vi "dfd_LatticeMA_Min_FIR_C.vi"() -> ()   [LabVIEW 2017, in "NI_DigFilterTemp.lvlib"]
uses:
  <vilib>/addons/Digital Filter Design/NI_DigFilterTemp.lvlib
panel:
  in  "String":string="\n\n/* ---- Constants ----*/\n#define %CapName%_N_COEFK %kCoefKAmt%\n#define %CapName%_N_STATES %CapName%_N_COEFK\n\n/* ---- Global Variables Declaration ----*/\nstatic %CoefAType% %FilterBlkName%_CoefK[%CapName%_N_COEFK];\n%InternalFunctionsDeclaration%\n\n%ShiftDefine%\n\n%AssistantFunctions%\n\n/* ---- Implement the Fixed-Point Filter ---- */ \n%OutType% %FilterBlkName%_Filtering (%InType% sampleIn, %FilterBlkName%_State state)\n{\n\tI32 accA, accB, accTmp;\n\t%MultType% mult;\n\tint i;\n\n\taccTmp = (%I32TypeCast%sampleIn << IN2DELAY);\n\taccA = (%I32TypeCast%sampleIn << IN2SUM);\n\t\n\tfor (i = 0; i < %CapName%_N_COEFK; i++)\n\t{\n\t\t/* Filtering */\n\t\tmult = %PreMultCast%(accA << SUM2MULT);\n\t\taccB = (%FilterBlkName%_%MultA%(mult, %FilterBlkName%_CoefK[i]) << PROD2SUM);\n\t\taccB += (state[i] << DELAY2SUM);\n\t\tmult = %PreMultCast%(state[i] << DELAY2MULT);\n\t\taccA += (%FilterBlkName%_%MultA%(mult, %FilterBlkName%_CoefK[i]) << PROD2SUM);\n\n\t\t/* Update the internal states */\n\t\tstate[i] = accTmp;\n\t\taccTmp = (accB << SUM2DELAY);\n\t}\n\n\t%ApplyGainAccA%\n\n\treturn (%OutType%)accA;\n}\n\n/* ---- Internal Functions ---- */\n%InternalFunctions%\n\n/* ---- Filter Coefficients ---- */\nstatic %CoefAType% %FilterBlkName%_CoefK [] = {\n%CoefficientsK%\n};\n"
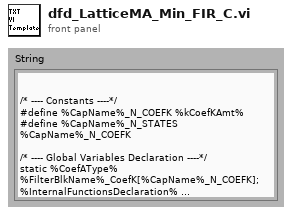
[diagram p1: front panel]
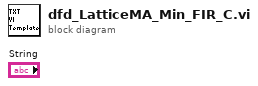
[diagram p0: block diagram]
diagram:
